vi "Eth Status Manager Close.vi"(8 "error in":errorcluster, 11 "Status Reference":T1) -> (0 "error out":errorcluster)   [LabVIEW 2019, in "Eth Status.lvlib"]
uses:
  Eth Status.lvlib
  Ctl/ICPCON Status.ctl
  MB_TCP2/MB_TCP_State.ctl
  MB_TCP2/MB_TCP.lvclass
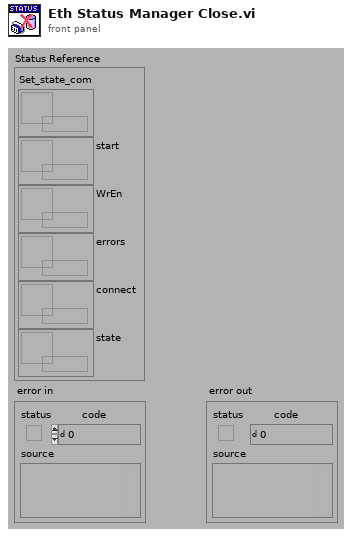
[diagram p1: front panel]
types:
  T1 = typedef "Eth Status.lvlib/ICPCON Status.ctl" = cluster{"Set_state_com":refnum<data-value>, "start":refnum<data-value>, "WrEn":refnum<data-value>, "errors":refnum<data-value>, "connect":refnum<data-value>, "state":refnum<data-value>}
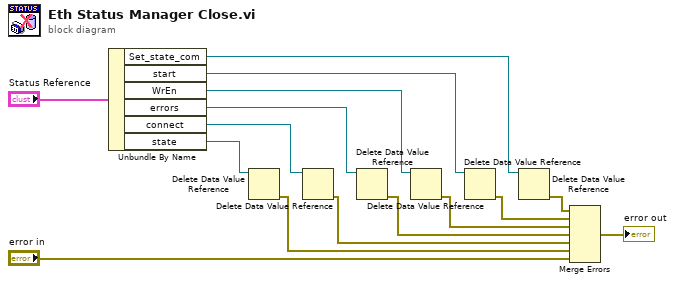
[diagram p0: block diagram]
diagram:
  n1 = Unbundle By Name("Status Reference") -> ("Set_state_com"=w7:refnum<data-value>, "start"=w15:refnum<data-value>, "WrEn"=w14:refnum<data-value>, "errors"=w13:refnum<data-value>, "connect"=w6:refnum<data-value>, "state"=w4:refnum<data-value>)
  n2 = Delete Data Value Reference(data value reference=w4) -> (error out=w3:errorcluster)  [unwired: 1 in, 1 out]
  n3 = Delete Data Value Reference(data value reference=w6) -> (error out=w5:errorcluster)  [unwired: 1 in, 1 out]
  n4 = Delete Data Value Reference(data value reference=w13) -> (error out=w11:errorcluster)  [unwired: 1 in, 1 out]
  n5 = Delete Data Value Reference(data value reference=w14) -> (error out=w12:errorcluster)  [unwired: 1 in, 1 out]
  n6 = Delete Data Value Reference(data value reference=w15) -> (error out=w9:errorcluster)  [unwired: 1 in, 1 out]
  n7 = Delete Data Value Reference(data value reference=w7) -> (error out=w8:errorcluster)  [unwired: 1 in, 1 out]
  n8 = Merge Errors(w8, w9, w12, w11, w5, w3, "error in") -> (→"error out":errorcluster)
